vi "Drive_Cheezy.vi"(3 "Joystick_In":T1) -> (0 "Right_Motor_Out":dbl, 1 "Left_Motor_Out":dbl)   [LabVIEW 2018]
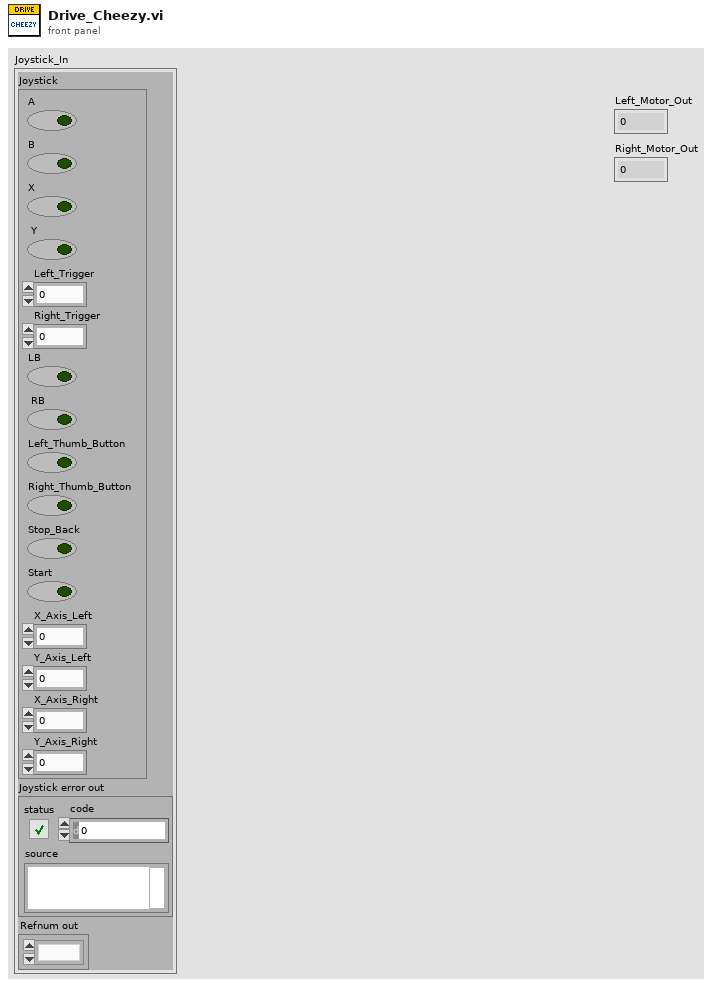
[diagram p1: front panel]
types:
  T1 = cluster{"Joystick":cluster{"A":bool, "B":bool, "X":bool, " Y":bool, "Left_Trigger":dbl, "Right_Trigger ":dbl, "LB":bool, " RB":bool, "Left_Thumb_Button":bool, "Right_Thumb_Button":bool, "Stop_Back":bool, "Start":bool, "X_Axis_Left":dbl, "Y_Axis_Left":dbl, "X_Axis_Right":dbl, "Y_Axis_Right":dbl}, "Joystick error out":errorcluster, "Refnum out":refnum<k1>}
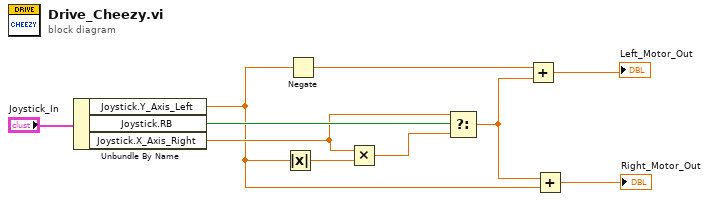
[diagram p0: block diagram]
diagram:
  n1 = Unbundle By Name("Joystick_In") -> ("Joystick.Y_Axis_Left"=w1:dbl, "Joystick.RB"=w5:bool, "Joystick.X_Axis_Right"=w3:dbl)
  n2 = Absolute Value(x=w1) -> (abs(x)=w4:dbl)
  n3 = Negate(x=w1) -> (-x=w9:dbl)
  n4 = Multiply(x=w3, y=w4) -> (x*y=w2:dbl)
  n5 = Select(t=w3, s=w5, f=w2) -> (s? t:f=w7:dbl)
  n6 = Add(x=w9, y=w7) -> (x+y=→"Left_Motor_Out":dbl)
  n7 = Add(x=w7, y=w1) -> (x+y=→"Right_Motor_Out":dbl)
